vi "自搭_姿态显示_故障注入1004.vi"() -> ()   [LabVIEW 2016]
uses:
  <vilib>/Instr/_visa.llb/VISA Configure Serial Port (Instr).vi
panel:
  out "命令显示":string
  in  "复位":bool
  in  "暂停":bool
  in  "小数":string
  in  "卡滞发生时间":string
  in  "角度（小数）":string
  in  "卡滞角度":string
  in  "退化故障":string(combo)
  in  "控制方法":string(combo)
  out "X":dbl(graph)
  out "Y":dbl(graph)
  in  "波特率":dbl
  in  "故障腿":string(combo)
  in  "data bits (8)":u16=8 caption="数据比特(8)" min=5 max=8 step=1
  in  "arduino端口":refnum<visa-resource-name>
  in  "控制程序启动":bool
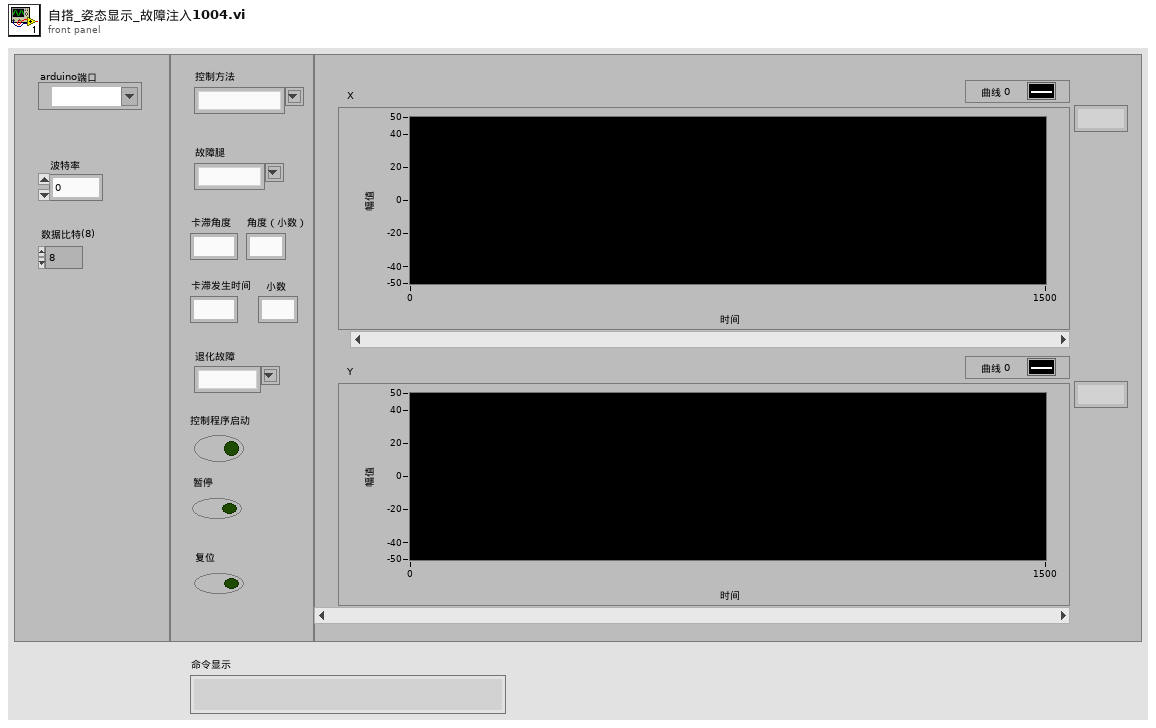
[diagram p1: front panel]
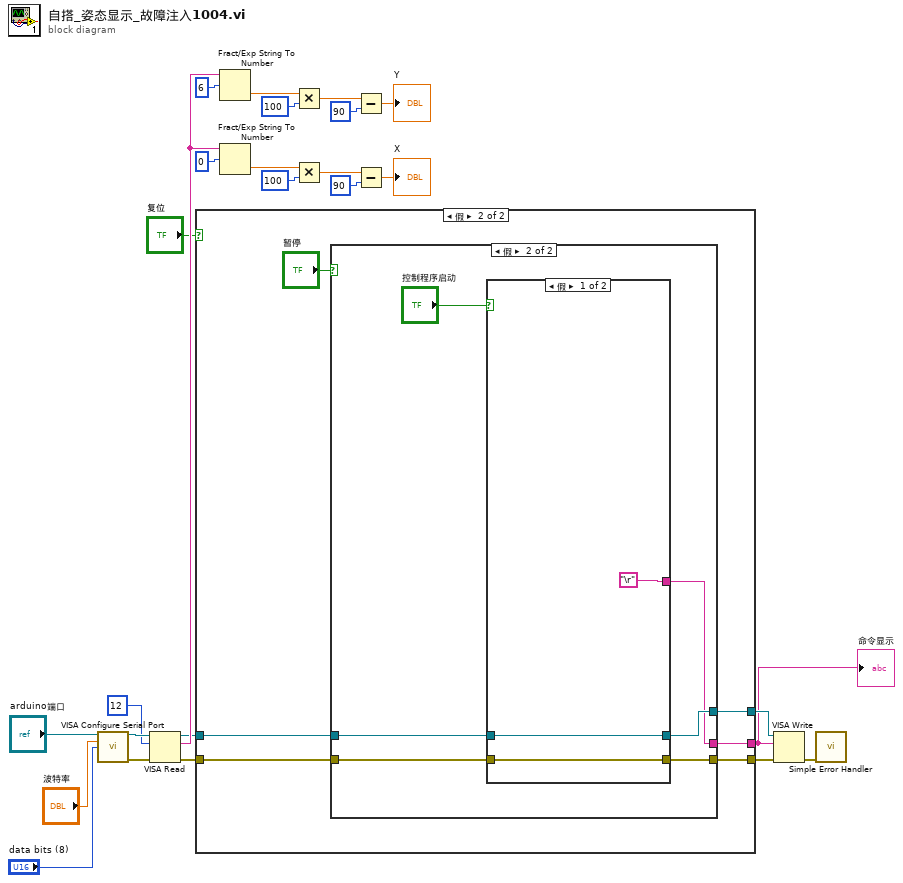
[diagram p0: block diagram]
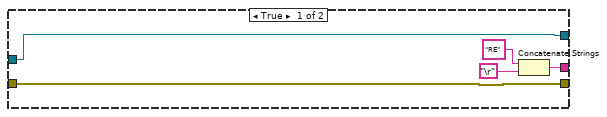
[diagram p2: hidden frame]
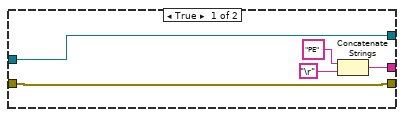
[diagram p3: hidden frame]
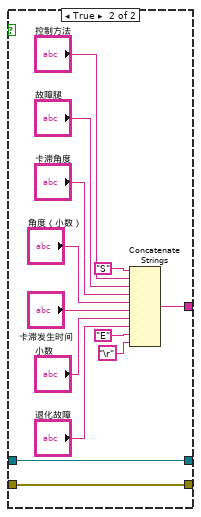
[diagram p4: hidden frame]
diagram:
  n1 = call-poly "VISA Configure Serial Port"("VISA resource name"="arduino端口", "baud rate (9600)"="波特率", "data bits (8)"="data bits (8)") -> ("VISA resource name out"=w23:refnum<visa-resource-name>, "error out"=w7:errorcluster)  [unwired: 11 in]
  n2 = VISA Read(VISA resource name=w23, byte count=12, error in (no error)=w7) -> (VISA resource name out=w8:refnum<visa-resource-name>, read buffer=w11:string, error out=w5:errorcluster)  [unwired: 1 out]
  n3 = case shown="假" "复位" {
    tunnel: w8 -> [w27 w37]
    tunnel: w5 -> [w28 w36]
    tunnel: [w27 w34] -> w3
    tunnel: [w29 w33] -> w1
    tunnel: [w28 w32] -> w2
    frame True {
      n4 = Concatenate Strings("RE", "\r") -> (w29:string)
    }
    frame False {
      n5 = case shown="假" "暂停" {
        tunnel: w37 -> [w40 w48]
        tunnel: w36 -> [w38 w46]
        tunnel: [w40 w45] -> w34
        tunnel: [w39 w44] -> w33
        tunnel: [w38 w43] -> w32
        frame True {
          n6 = Concatenate Strings("PE", "\r") -> (w39:string)
        }
        frame False {
          n7 = case shown="假" "控制程序启动" {
            tunnel: w48 -> [w50 w54]
            tunnel: w46 -> [w51 w52]
            tunnel: [w50 w54] -> w45
            tunnel: ["\r" w53] -> w44
            tunnel: [w51 w52] -> w43
            frame False {
            }
            frame True {
              n8 = Concatenate Strings("S", "控制方法", "故障腿", "卡滞角度", "角度（小数）", "卡滞发生时间", "小数", "退化故障", "E", "\r") -> (w53:string)
            }
          }
        }
      }
    }
  }
  "命令显示" <- w1
  n9 = Fract/Exp String To Number(string=w11, offset=6) -> (number=w15:dbl)  [unwired: 3 out]
  n10 = Fract/Exp String To Number(string=w11, offset=0) -> (number=w20:dbl)  [unwired: 3 out]
  n11 = Multiply(x=w15, y=100) -> (x*y=w13:dbl)
  n12 = Multiply(x=w20, y=100) -> (x*y=w18:dbl)
  n13 = Subtract(x=w13, y=90) -> (x-y=→"Y":dbl)
  n14 = Subtract(x=w18, y=90) -> (x-y=→"X":dbl)
  n15 = VISA Write(VISA resource name=w3, write buffer=w1, error in (no error)=w2) -> (error out=w4:errorcluster)  [unwired: 2 out]
  n16 = call <vilib>:"Simple Error Handler.vi"("error in (no error)"=w4) -> ()  [unwired: 1 in, 8 out]
